vi "Day1.vi"() -> ()   [LabVIEW 2024]
uses:
  <vilib>/Utility/file.llb/Read Delimited Spreadsheet (I64).vi
panel:
  out "sum":i64
  out "Array":i64[][](array[numeric])
  out "all rows":i64[][](array[numeric])
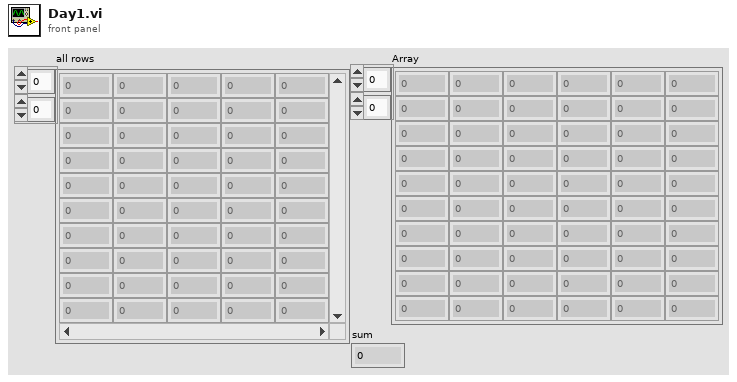
[diagram p1: front panel]
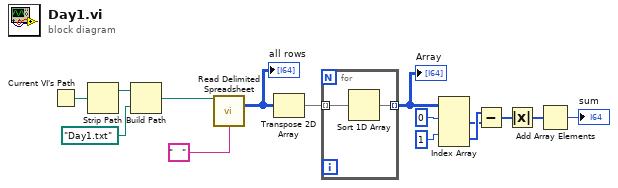
[diagram p0: block diagram]
diagram:
  n1 = Current VI's Path() -> (path=w15:path)
  n2 = Strip Path(path=w15) -> (stripped path=w14:path)  [unwired: 1 out]
  n3 = Build Path(base path=w14, name or relative path=path "Day1.txt") -> (appended path=w12:path)
  n4 = call-poly <vilib>:"Read Delimited Spreadsheet.vi"("file path (dialog if empty)"=w12, "delimiter (\\t)"="   " ("delimiter (\\t)")) -> ("all rows"=w10:i64[][])  [unwired: 8 in, 5 out]
  "all rows" <- w10
  n5 = Transpose 2D Array(2D array=w10) -> (transposed array=w9:i64[][])
  n6 = for {
    tunnel: w9 -> [w17] mode=indexing
    tunnel: [w16] -> w8 mode=indexing
    n7 = Sort 1D Array(array=w17) -> (sorted array=w16:i64[])
  }
  "Array" <- w8
  n8 = Index Array(array=w8, index (row) #1=0 ("index (row)"), index (row) #2=1 ("index (row)")) -> (element #1=w4:i64[], element #2=w5:i64[])  [unwired: 2 in]
  n9 = Subtract(x=w5, y=w4) -> (x-y=w3:i64[])
  n10 = Absolute Value(x=w3) -> (abs(x)=w2:i64[])
  n11 = Add Array Elements(numeric array=w2) -> (sum=→"sum":i64)
